vi "Get Comm Connections.vi"(8 "error in (no error)":errorcluster, 11 "VeriStand Comm in":refnum<class "VeriStand Comm.lvclass">) -> (0 "error out":errorcluster, 2 "Number of Connections":i32, 3 "VeriStand Comm out":refnum<class "VeriStand Comm.lvclass">)   [LabVIEW 2027, in "NI VeriStand Addon Network Comm.lvlib" / "VeriStand Comm.lvclass"]
uses:
  VeriStand Comm.lvclass
  <vilib>/NI/STM/Connection Manager/TCP/TCP Connection Method.ctl
  VeriStand Comm.lvclass/VeriStand Comm.ctl
  <vilib>/NI/STM/SubVIs/Generate STM Error.vi
  <vilib>/NI/STM/NI STM.lvlib
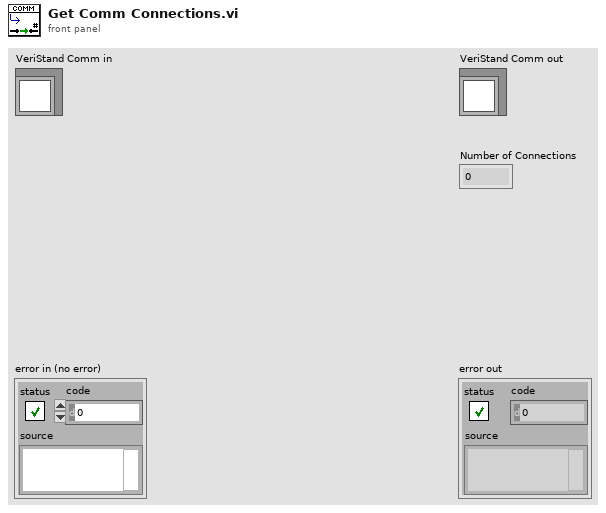
[diagram p1: front panel]
types:
  T1 = typedef "NI STM.lvlib/TCP Connection Method.ctl" = enum16{"Initialize", "Add Connection", "Set Properties", "Get Connection(s)", "Remove Connection", "Remove All Connections", "Get Connection Count"}
  T2 = typedef "NI STM.lvlib/TCP Connection Manager Reference.ctl" = refnum<data-value>
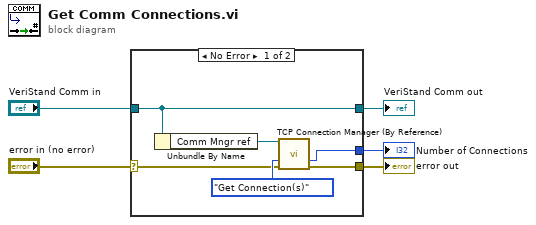
[diagram p0: block diagram]
diagram:
  n1 = case shown="No Error" "error in (no error)" {
    selector: "error in (no error)" -> [w7 w13]
    tunnel: [w6 w13] -> w4
    tunnel: [w11 w12] -> w2
    tunnel: "VeriStand Comm in" -> [w11 w12]
    tunnel: [w8 _] -> w1
    frame No Error {
      n2 = Unbundle By Name(w11) -> ("Comm Mngr ref"=w9:T2)
      n3 = call <vilib>:"TCP Connection Manager (By Reference).vi"("connection manager ref in"=w9, "method"=TCP_Connection_Method."Get Connection(s)", "error in"=w7) -> ("number of connections"=w8:i32, "error out"=w6:errorcluster)  [unwired: 6 in, 5 out]
    }
    frame Error {
    }
  }
  "error out" <- w4
  "VeriStand Comm out" <- w2
  "Number of Connections" <- w1
